vi "CustomersData_Create.vi"(0 "reference in":refnum<class "CustomersData.lvclass">, 2 "StringRef":refnum<vi>, 5 "error in (no error)":errorcluster) -> (14 "reference out":refnum<class "CustomersData.lvclass">, 19 "error out":errorcluster)   [LabVIEW 2020, in "CustomersData.lvclass"]
uses:
  CustomersData.lvclass
  C:/Projects/DesignPatterns/Bridge1/DataObject_class/DataObject.lvclass
  DataObject_class/DataObject.lvclass
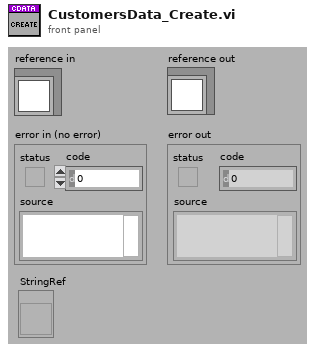
[diagram p1: front panel]
types:
  T1 = typedef "CustomersData.lvclass/ObjectAttributes.ctl" = cluster{"_customers":string[], "_current":i32}
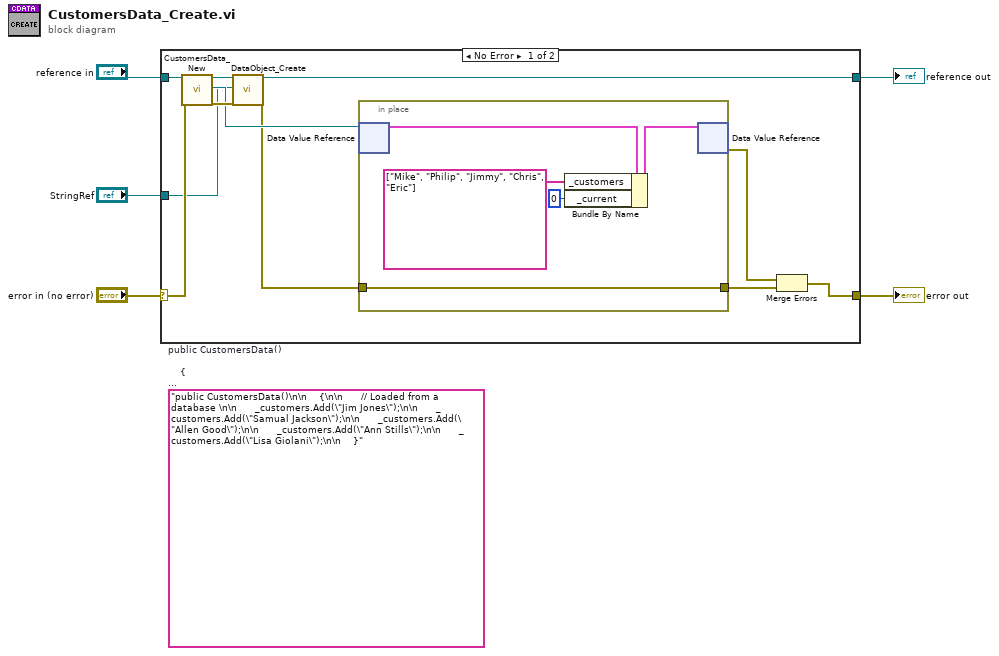
[diagram p0: block diagram]
diagram:
  (unwired) "public CustomersData()\n\n    {\n\n      // Loaded from a database \n\n      _customers.Add(\"Jim Jones\");\n\n      _customers.Add(\"Samual Jackson\");\n\n      _customers.Add(\"Allen Good\");\n\n      _customers.Add(\"Ann Stills\");\n\n      _customers.Add(\"Lisa Giolani\");\n\n    }"  # public CustomersData()      {        // Loaded from a database         _customers.Add("Jim Jones");        _customers.Add("Samual Jackson");        _customers.Add("Allen Good");        _customers.Add("Ann Stills");        _customers.Add("Lisa Giolani");      }
  n1 = case shown="No Error" "error in (no error)" {
    selector: "error in (no error)" -> [w15 w23]
    tunnel: [w13 w23] -> w4
    tunnel: "reference in" -> [w16 w22]
    tunnel: [w10 w22] -> w2
    tunnel: "StringRef" -> [w6 _]
    frame No Error {
      n2 = call "CustomersData_New.vi"("reference in"=w16, "error in (no error)"=w15) -> ("reference out"=w12:refnum<class "CustomersData.lvclass">, "DVRRefOut"=w9:refnum<data-value>, "error out"=w11:errorcluster)  [unwired: 14 in, 1 out]
      n3 = call "DataObject_Create.vi"("reference in"=w12, "StringRef"=w6, "error in (no error)"=w11) -> ("reference out"=w10:refnum<class "CustomersData.lvclass">, "error out"=w8:errorcluster)  [unwired: 15 in]
      n4 = in-place {
        in-place-border: w8 -> [w19]
        in-place-border: [w19] -> w7
        n5 = in-place-dvr #1(w9) -> (w20:T1)  [unwired: 1 out]
        n6 = Bundle By Name(cluster=w20, "_customers"=string[] ["Mike", "Philip", "Jimmy", "Chris", "Eric"], "_current"=0) -> (w21:T1)
        n7 = in-place-dvr #1(w21) -> (w14:errorcluster)  [unwired: 1 out]
      }
      n8 = Merge Errors(w14, w7) -> (w13:errorcluster)
    }
    frame Error {
    }
  }
  "error out" <- w4
  "reference out" <- w2
